vi "RefreshGraphArr.vi"(8 "error in (no error)":errorcluster caption="entrée d'erreur (pas d'erreur)", 11 "Interface en entrée":refnum<class "Interface.lvclass"> caption="DNL_LabVIEW Object in") -> (0 "error out":errorcluster caption="sortie d'erreur", 3 "Interface en sortie":refnum<class "Interface.lvclass"> caption="DNL_LabVIEW Object out")   [LabVIEW 2019, in "Interface.lvclass"]
uses:
  Interface.lvclass
  Interface.lvclass/Interface.ctl
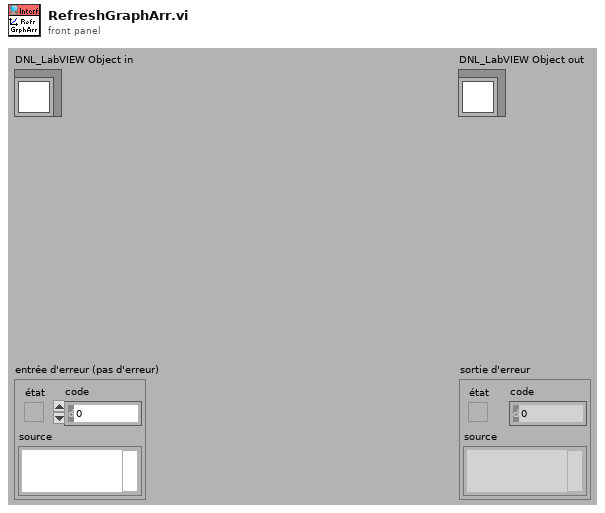
[diagram p1: front panel]
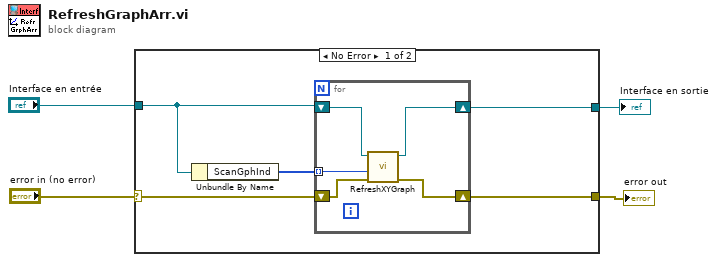
[diagram p0: block diagram]
diagram:
  n1 = case shown="No Error" "error in (no error)" {
    selector: "error in (no error)" -> [w8 w16]
    tunnel: [w7 w16] -> w3
    tunnel: [w5 w15] -> w1
    tunnel: "Interface en entrée" -> [w6 w15]
    frame No Error {
      n2 = Unbundle By Name(w6) -> ("ScanGphInd"=w9:i32[])
      n3 = for {
        shift-right: [w13] -> w7
        shift-left: w8 -> [w14]
        tunnel: w9 -> [w10] mode=indexing
        shift-right: [w11] -> w5
        shift-left: w6 -> [w12]
        n4 = call "RefreshXYGraph.vi"("error in (no error)"=w14, "Graph Index"=w10, "Interface en entrée"=w12) -> ("error out"=w13:errorcluster, "Interface en sortie"=w11:refnum<class "Interface.lvclass">)  [unwired: 6 in, 1 out]
      }
    }
    frame Error {
    }
  }
  "error out" <- w3
  "Interface en sortie" <- w1
